vi "TcpSendData.vi"(8 "error in (no error)":errorcluster, 10 "Pound in":refnum<class "Pound.lvclass">, 11 "Qbus in":refnum<class "Qbus.lvclass">) -> (0 "error out":errorcluster)   [LabVIEW 2017, in "ServerComm.lvlib"]
uses:
  <vilib>/addons/InsightCM/Devices/Shared/Common/ServerComm/ServerComm.lvlib
  <vilib>/addons/Qbus/Qbus.lvclass
  <vilib>/NI/Software Watchdog/Pound/Pound.lvclass
  <vilib>/addons/InsightCM/Devices/Shared/Common/ServerComm/controls/TcpSendDataConfig.ctl
  <vilib>/addons/InsightCM/Devices/Shared/Common/ServerComm/controls/DataSendParameters.ctl
  <vilib>/addons/TraceLogger/TraceLogger.lvlib
  <vilib>/NI/Software Watchdog/Watchdog/Watchdog.lvclass
  <vilib>/addons/InsightCM/Utilities/GlobalConfiguration/GlobalConfiguration.lvlib
  <vilib>/addons/InsightCM/Utilities/PropertyHelpers/PropertyHelpers.lvlib
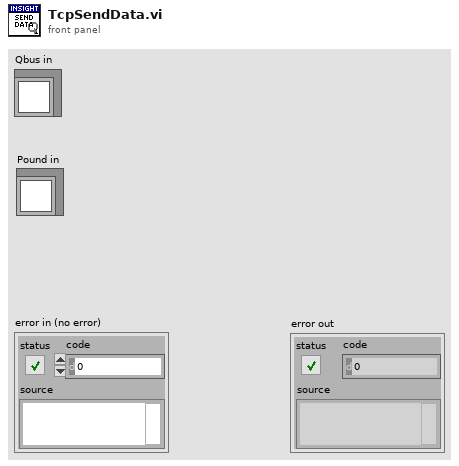
[diagram p1: front panel]
types:
  T1 = typedef "ServerComm.lvlib/TcpSendDataConfig.ctl" = cluster{"SendParams":T2}
  T2 = typedef "ServerComm.lvlib/DataSendParameters.ctl" = cluster{"PacketSizeKbytes":i32, "InterPacketDelay":i32}
  T3 = typedef "SectionKeyValues.ctl" = cluster{"Section":string, "KeyValues":T4[]}
  T4 = typedef "KeyValuePair.ctl" = cluster{"Key":string, "Value":string}
  T5 = typedef "ServerComm.lvlib/DataSendBody.ctl" = cluster{"tcp reference":T6, "SendFileMode":T7, "data":variant, "IRoutingSource":T8, "ReplyTo":string}
  T6 = typedef "TcpMessageReference.ctl" = refnum<data-value>
  T7 = typedef "ServerComm.lvlib/DataSendMode.ctl" = enum16{"File", "InMemoryFile", "Stream", "StreamFileBlock", "ByteArray", "NoOp", "UnknownData"}
  T8 = typedef "IRoutingSource.ctl" = cluster{"CorrelationId":string, "ReplyTo":string}
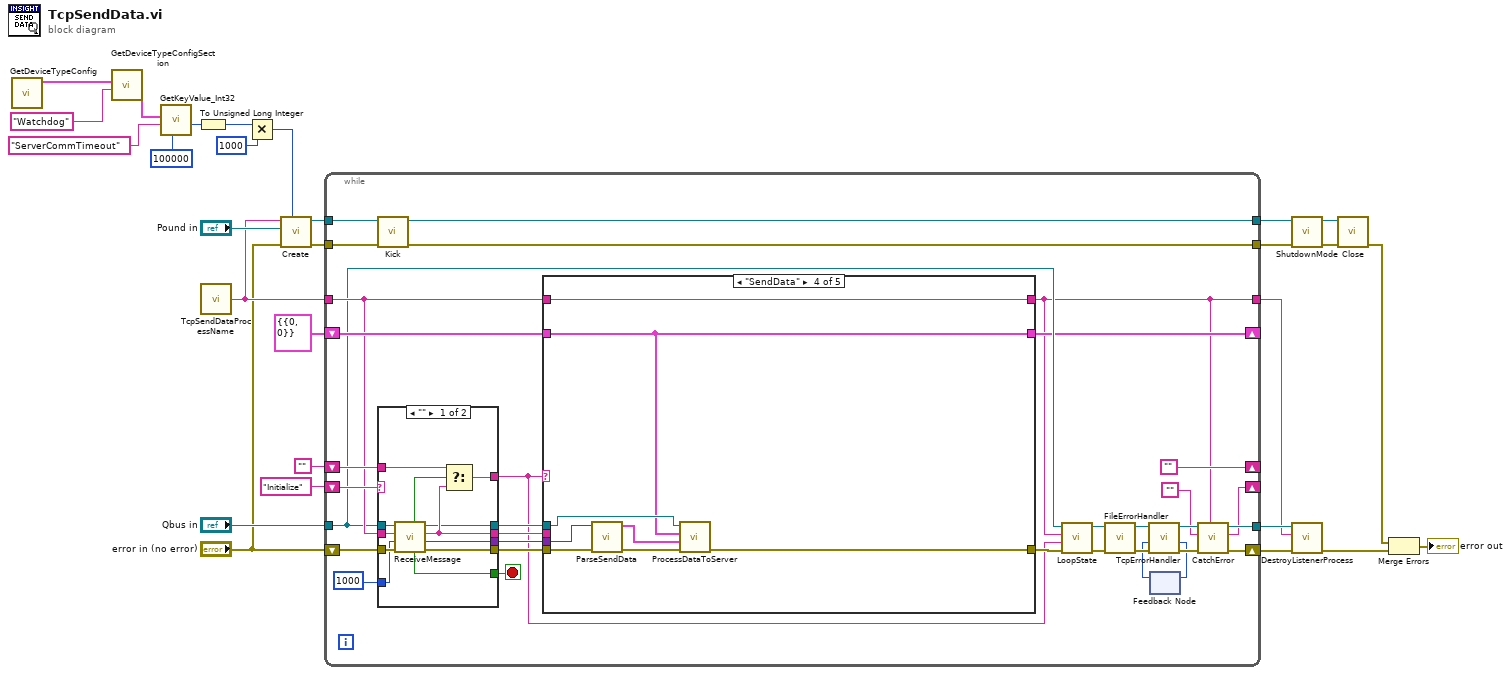
[diagram p0: block diagram]
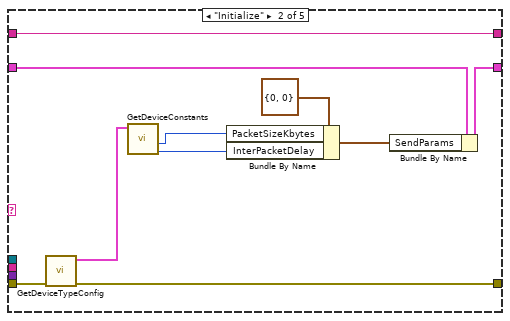
[diagram p4: hidden frame]
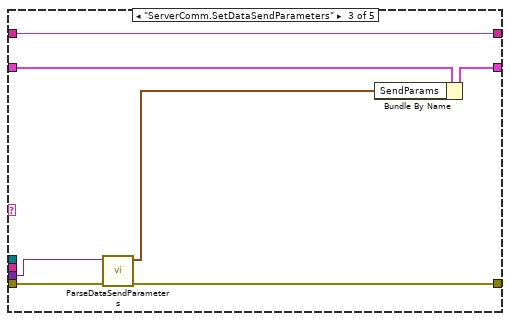
[diagram p5: hidden frame]
diagram:
  n1 = call <vilib>:"GetDeviceTypeConfig.vi"() -> ("key values"=w9:T3[])  [unwired: 9 in, 2 out]
  n2 = call <vilib>:"GetDeviceTypeConfigSection.vi"("key"="Watchdog", "key values"=w9) -> ("key value pairs out"=w7:T4[])  [unwired: 8 in, 1 out]
  n3 = call <vilib>:"GetKeyValue_Int32.vi"("default"=100000 ("Execution Timeout (ms)"), "key"="ServerCommTimeout" ("Tag"), "key value pairs"=w7) -> ("value"=w5:i32)  [unwired: 6 in, 2 out]
  n4 = To Unsigned Long Integer(number=w5) -> (unsigned 32bit integer=w2:u32)
  n5 = call <vilib>:"TcpSendDataProcessName.vi"() -> ("process name"=w11:string)  [unwired: 5 in]
  n6 = Multiply(x=w2, y=u32 1000) -> (x*y=w1:u32)
  n7 = call <vilib>:"Create.vi"("Execution Timeout (ms)"=w1, "error in (no error)"="error in (no error)", "Pound"="Pound in", "Name"=w11) -> ("error out"=w12:errorcluster, "Watchdog"=w13:refnum<data-value>)  [unwired: 6 in]
  n8 = while {
    shift-right: [""] -> _
    shift-left: "" -> [w60]
    tunnel: "Qbus in" -> [w44]
    tunnel: w11 -> [w45]
    tunnel: [w49] -> w26
    tunnel: [w32] -> w25
    shift-right: [w47] -> _
    shift-left: "Initialize" -> [w54]
    shift-right: [w41] -> _
    shift-left: T1 {"SendParams"={"PacketSizeKbytes"=0, "InterPacketDelay"=0}} ("config") -> [w53]
    tunnel: [w40] -> w15
    tunnel: [w39] -> w14
    tunnel: w13 -> [w38]
    tunnel: w12 -> [w37]
    shift-right: [w51] -> w27
    shift-left: "error in (no error)" -> [w42]
    stop <- w61 stop-if-true
    n9 = call <vilib>:"Kick.vi"("error in (no error)"=w37, "Watchdog"=w38) -> ("error out"=w39:errorcluster, "Watchdog"=w40:refnum<data-value>)  [unwired: 8 in]
    n10 = case shown="\"\"" w54 {
      selector: w54 -> [_ w74]
      tunnel: w42 -> [w64 w76]
      tunnel: [w70 w76] -> w59
      tunnel: [w69 _] -> w55
      tunnel: [w65 _] -> w61
      tunnel: [w68 _] -> w56
      tunnel: w60 -> [w73 _]
      tunnel: [w72 w74] -> w43
      tunnel: [w67 w75] -> w57
      tunnel: 1000 ("milliseconds to wait") -> [w63 _]
      tunnel: w44 -> [w66 w75]
      tunnel: w45 -> [w62 _]
      frame "" {
        n11 = call <vilib>:"ReceiveMessage.vi"("error in (no error)"=w64, "timeout (0)"=w63, "process name"=w62, "Qbus in"=w66) -> ("error in (no error)"=w70:errorcluster, "message value"=w69:variant, "message name"=w68:string, "Qbus out"=w67:refnum<class "Qbus.lvclass">, "exit"=w65:bool, "timed out"=w71:bool)  [unwired: 2 in]
        n12 = Select(t=w73, s=w71, f=w68) -> (s? t:f=w72:string)
      }
      frame Default {
      }
    }
    n13 = case shown="\"SendData\"" w43 {
      tunnel: w59 -> [w78 w84 w94 w104 w105]
      tunnel: w57 -> [_ _ _ w100 _]
      tunnel: [w78 w83 w93 w98 w105] -> w46
      tunnel: w56 -> [_ _ _ _ _]
      tunnel: w55 -> [_ _ w92 w103 _]
      tunnel: w53 -> [w79 w86 w96 w99 w107]
      tunnel: [w79 w85 w95 w99 w107] -> w41
      tunnel: w45 -> [w77 w89 w90 w97 w106]
      tunnel: [w77 w89 w90 w97 w106] -> w32
      frame "", Default {
      }
      frame "Initialize" {
        n14 = call <vilib>:"GetDeviceTypeConfig.vi"("error in (no error)"=w84) -> ("error out"=w83:errorcluster, "key values"=w82:T3[])  [unwired: 8 in, 1 out]
        n15 = call <vilib>:"GetDeviceConstants.vi"("key values"=w82) -> ("InterPacketDelay"=w80:i32, "PacketSizeKbyte"=w81:i32)  [unwired: 7 in, 2 out]
        n16 = Bundle By Name(cluster=T2 {"PacketSizeKbytes"=0, "InterPacketDelay"=0} ("SendParams"), "PacketSizeKbytes"=w81, "InterPacketDelay"=w80) -> (w88:T2)
        n17 = Bundle By Name(cluster=w86, "SendParams"=w88) -> (w85:T1)
      }
      frame "ServerComm.SetDataSendParameters" {
        n18 = call <vilib>:"ParseDataSendParameters.vi"("error in (no error)"=w94, "body"=w92) -> ("error out"=w93:errorcluster, "data send parameters"=w91:T2)  [unwired: 8 in]
        n19 = Bundle By Name(cluster=w96, "SendParams"=w91) -> (w95:T1)
      }
      frame "SendData" {
        n20 = call <vilib>:"ParseSendData.vi"("error in (no error)"=w104, "body"=w103) -> ("error out"=w102:errorcluster, "data send"=w101:T5)  [unwired: 8 in]
        n21 = call <vilib>:"ProcessDataToServer.vi"("error in (no error)"=w102, "data send"=w101, "config"=w99, "qbus in"=w100) -> ("error out"=w98:errorcluster)  [unwired: 7 in]
      }
      frame "Exit" {
      }
    }
    n22 = call <vilib>:"LoopState.vi"("error in (no error)"=w46, "loop action"=w43, "process name"=w32, "Qbus in"=w44) -> ("error out"=w36:errorcluster, "Qbus out"=w34:refnum<class "Qbus.lvclass">)  [unwired: 6 in]
    n23 = call <vilib>:"FileErrorHandler.vi"("error in (no error)"=w36, "Qbus in"=w34) -> ("error out"=w35:errorcluster, "Qbus out"=w33:refnum<class "Qbus.lvclass">)  [unwired: 8 in]
    n24 = feedback #1() -> (w29:i32)  [unwired: 1 in]
    n25 = call <vilib>:"TcpErrorHandler.vi"("error in (no error)"=w35, "consequtive error count in"=w29, "Qbus in"=w33) -> ("error out"=w52:errorcluster, "consequtive error count out"=w30:i32, "Qbus out"=w50:refnum<class "Qbus.lvclass">)  [unwired: 6 in]
    n26 = feedback-in #1(w30) -> ()
    n27 = call <vilib>:"CatchError.vi"("source"=w32, "error in (no error)"=w52, "next action in"="", "Qbus in"=w50) -> ("error out"=w51:errorcluster, "next action out"=w47:string, "Qbus out"=w49:refnum<class "Qbus.lvclass">)  [unwired: 5 in]
  }
  n28 = call <vilib>:"ShutdownMode.vi"("error in (no error)"=w14, "Watchdog"=w15) -> ("error out"=w20:errorcluster, "Watchdog"=w21:refnum<data-value>)  [unwired: 8 in]
  n29 = call <vilib>:"DestroyListenerProcess.vi"("error in (no error)"=w27, "process name"=w25, "Qbus in"=w26) -> ("error in (no error)"=w18:errorcluster)  [unwired: 7 in, 1 out]
  n30 = call <vilib>:"Close.vi"("error in (no error)"=w20, "Watchdog"=w21) -> ("error out"=w19:errorcluster)  [unwired: 9 in]
  n31 = Merge Errors(w19, w18) -> (→"error out":errorcluster)
